vi "Connection Generator.vi"() -> ()   [LabVIEW 2019]
uses:
  <vilib>/numeric/Random Number (Range) I64.vi
  <vilib>/numeric/sub_Random U32.vi
panel:
  out "bytes written":i32
  out "error out (no error) 2":errorcluster
  in  "error in (no error)":errorcluster
  out "T1A1/A2":bool
  out "T1A13/A14":bool
  out "T1A11/A12":bool
  out "T1A9/A10":bool
  out "T1A8":bool
  out "T1A7":bool
  out "T1A5/A6":bool
  out "T1A3/A4":bool
  out "T1F3":bool
  out "T1F1/F2":bool
  out "T1E13/E14":bool
  out "T1E11/E12":bool
  out "T1E9/E10":bool
  out "T1E8":bool
  out "T1E7":bool
  out "T1E5":bool
  out "T1E3/E4":bool
  out "T1E1/E2":bool
  out "T1D13/D14":bool
  out "T1D11/D12":bool
  out "T1D9/D10":bool
  out "T1D8":bool
  out "T1D7":bool
  out "T1D5/D6":bool
  out "T1D3/D4":bool
  out "T1D1/D2":bool
  out "T1C13/C14":bool
  out "T1C11/C12":bool
  out "T1C9/C10":bool
  out "T1C8":bool
  out "T1C7":bool
  out "T1C5/C6":bool
  out "T1C3/C4":bool
  out "T1C1/C2":bool
  out "T1B13/B14":bool
  out "T1B11/B12":bool
  out "T1B9/B10":bool
  out "T1B8":bool
  out "T1B7":bool
  out "T1B5/B6":bool
  out "T1B3/B4":bool
  out "T1B1/B2":bool
  out "T2A1/A2":bool
  out "T2A13/A13":bool
  out "T2A11/A12":bool
  out "T2A9/A10":bool
  out "T2A8":bool
  out "T2A7":bool
  out "T2A5/A6":bool
  out "T2A3/A4":bool
  out "T2G5/G6":bool
  out "T2G3/G4":bool
  out "T2G1/G2":bool
  out "T2F6/F7":bool
  out "T2F4/F5":bool
  out "T2F3":bool
  out "T2F1/F2":bool
  out "T2E13/E14":bool
  out "T2E11/E12":bool
  out "T2E9/E10":bool
  out "T2E8":bool
  out "T2E7":bool
  out "T2E5/E6":bool
  out "T2E3/E4":bool
  out "T2E1/E2":bool
  out "T2D13/D14":bool
  out "T2D11/D12":bool
  out "T2D9/D10":bool
  out "T2D8":bool
  out "T2D7":bool
  out "T2D5/D6":bool
  out "T2D3/D4":bool
  out "T2D1/D2":bool
  out "T2C13/C14":bool
  out "T2C11/C12":bool
  out "T2C9/C10":bool
  out "T2C8":bool
  out "T2C7":bool
  out "T2C5/C6":bool
  out "T2C3/C4":bool
  out "T2C1/C2":bool
  out "T2B13/B14":bool
  out "T2B11/B12":bool
  out "T2B9/B10":bool
  out "T2B8":bool
  out "T2B7":bool
  out "T2B5/B6":bool
  out "T2B3/B4":bool
  out "T2B1/B2":bool
  out "I3":bool
  out "I2":bool
  out "I1":bool
  out "T3H6":bool
  out "T3H4":bool
  out "T3H3":bool
  out "T3H1":bool
  out "T3G13/G14":bool
  out "T3G11/G12":bool
  out "T3G9/G10":bool
  out "T3G8":bool
  out "T3G7":bool
  out "T3G5/G6":bool
  out "T3G3/G4":bool
  out "T3G1/G2":bool
  out "T3F13/F14":bool
  out "T3F11/F12":bool
  out "T3F9/F10":bool
  out "T3F8":bool
  out "T3F7":bool
  out "T3F5/F6":bool
  out "T3F3/F4":bool
  out "T3F1/F2":bool
  out "T3E13/E14":bool
  out "T3E11/E12":bool
  out "T3E9/E10":bool
  out "T3E8":bool
  out "T3E7":bool
  out "T3E5/E6":bool
  out "T3E3/E4":bool
  out "T3E1/E2":bool
  out "T3D13/D14":bool
  out "T3D11/D12":bool
  out "T3D9/D10":bool
  out "T3D8":bool
  out "T3D7":bool
  out "T3D5/D6":bool
  out "T3D3/D4":bool
  out "T3D1/D2":bool
  out "T3C13/C14":bool
  out "T3C11/C12":bool
  out "T3C9/C10":bool
  out "T3C8":bool
  out "T3C7":bool
  out "T3C5/C6":bool
  out "T3C3/C4":bool
  out "T3C1/C2":bool
  out "T3B13/B14":bool
  out "T3B11/B12":bool
  out "T3B9/B10":bool
  out "T3B8":bool
  out "T3B7":bool
  out "T3B5/B6":bool
  out "T3B3/B4":bool
  out "T3B1/B2":bool
  out "T3A13/A14":bool
  out "T3A11/A12":bool
  out "T3A9/A10":bool
  out "T3A8":bool
  out "T3A7":bool
  out "T3A5/A6":bool
  out "T3A3/A4":bool
  out "T3A1/A2":bool
  in  "Stop":bool
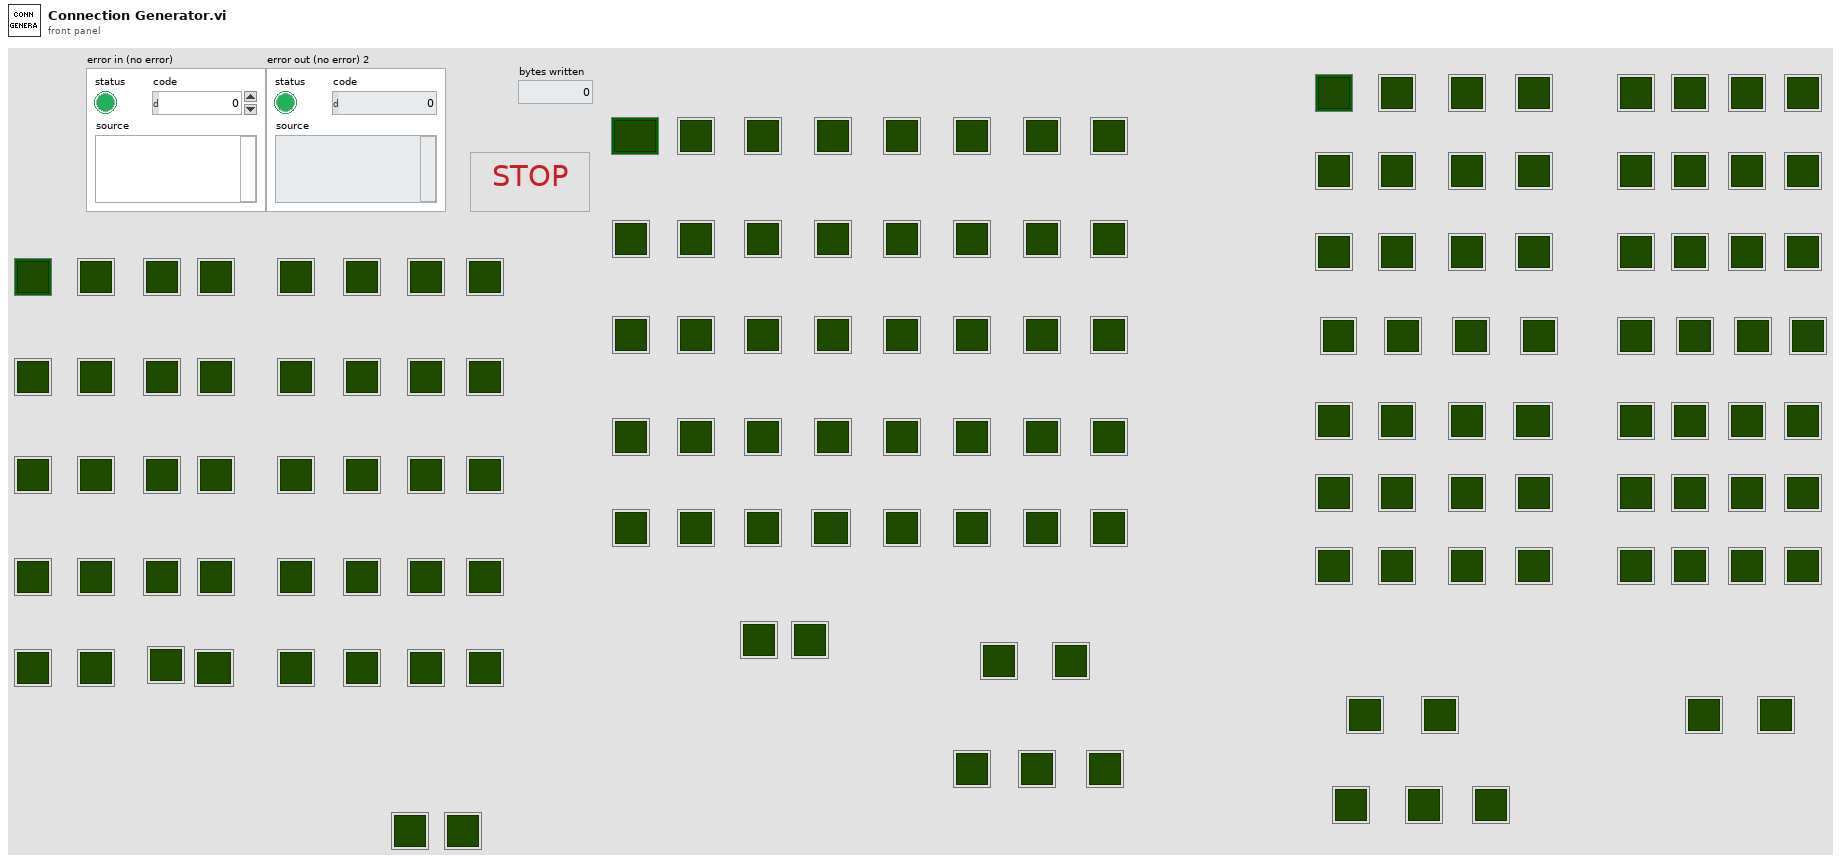
[diagram p1: front panel]
types:
  T1 = enum16{"Initialize", "Create Random String", "Open Connection", "Send Data", "Close Connection", "Exit"}
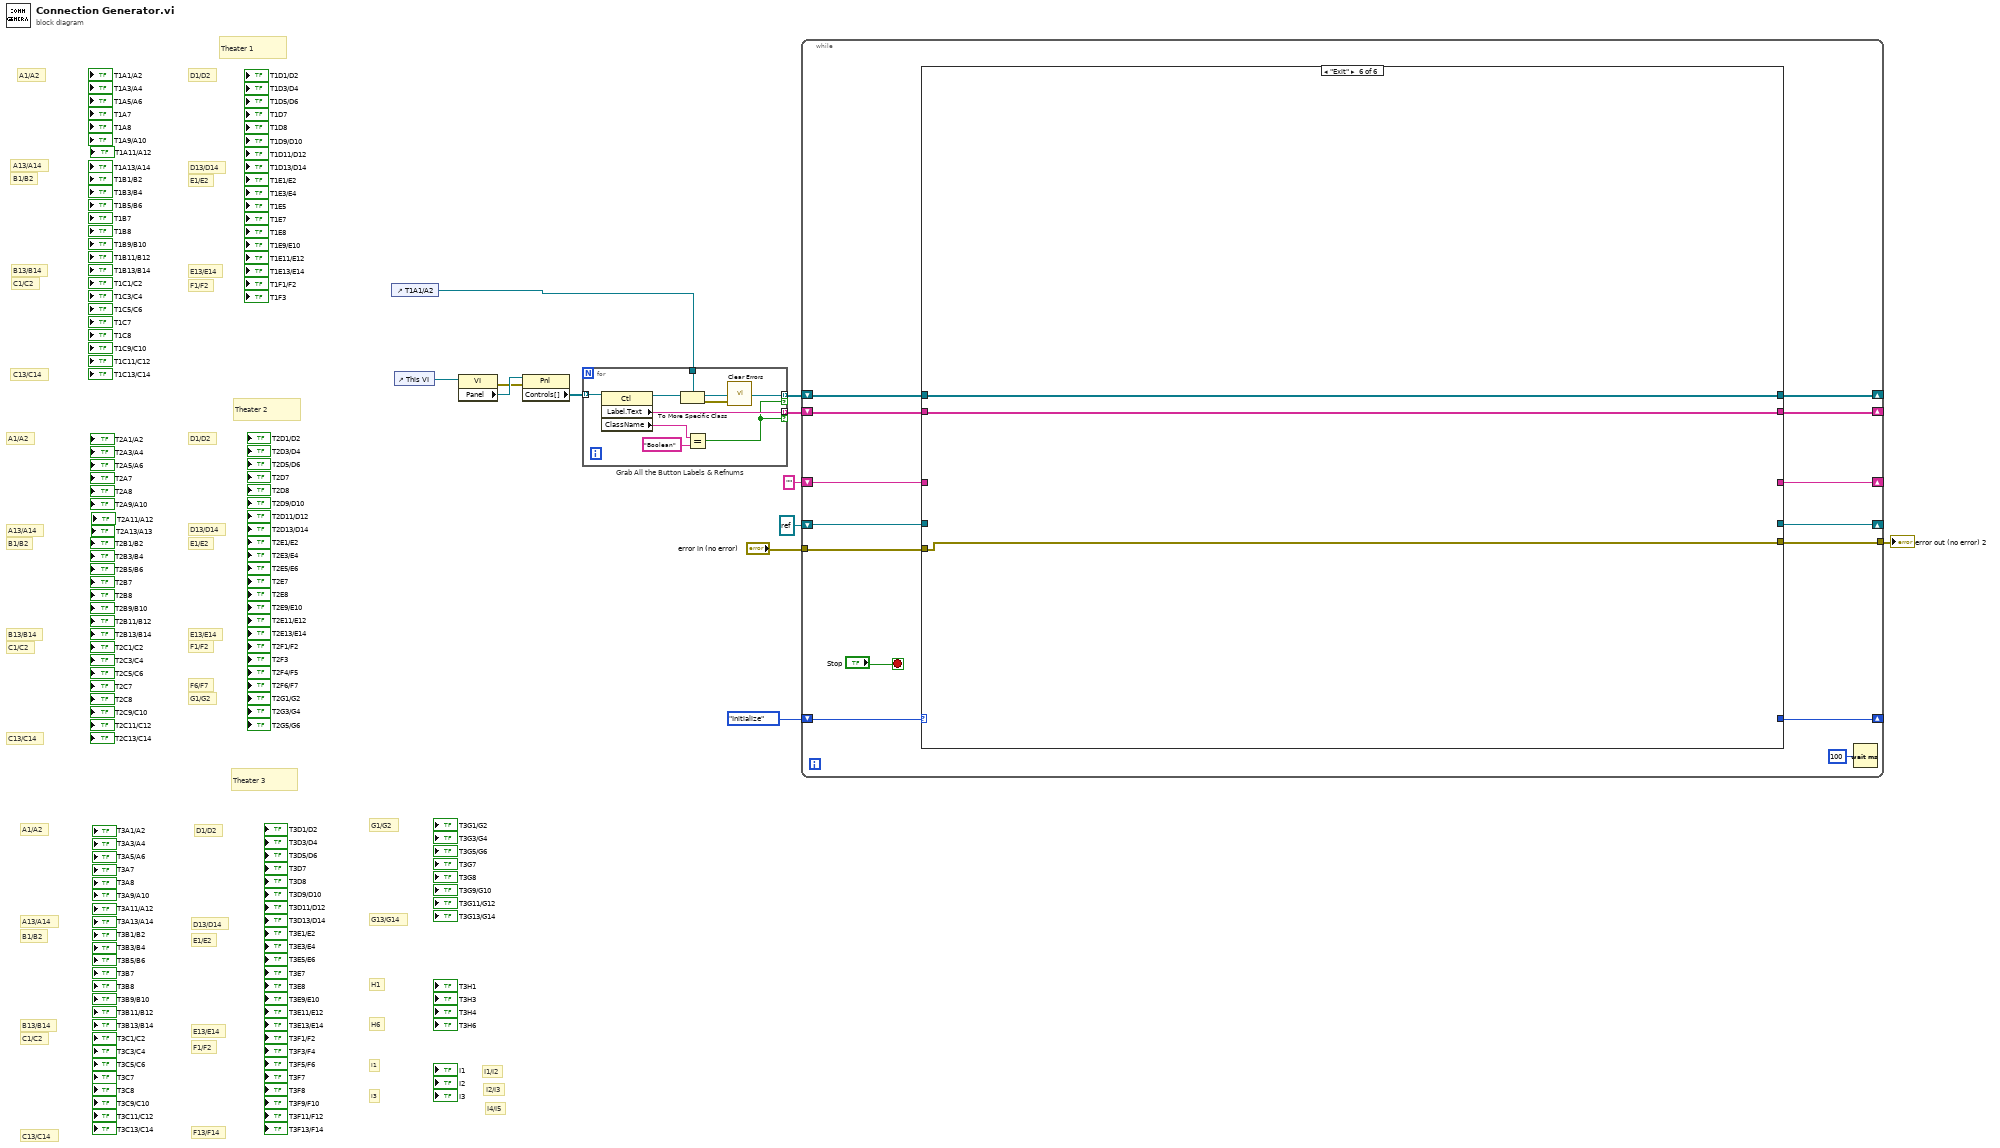
[diagram p0: block diagram]
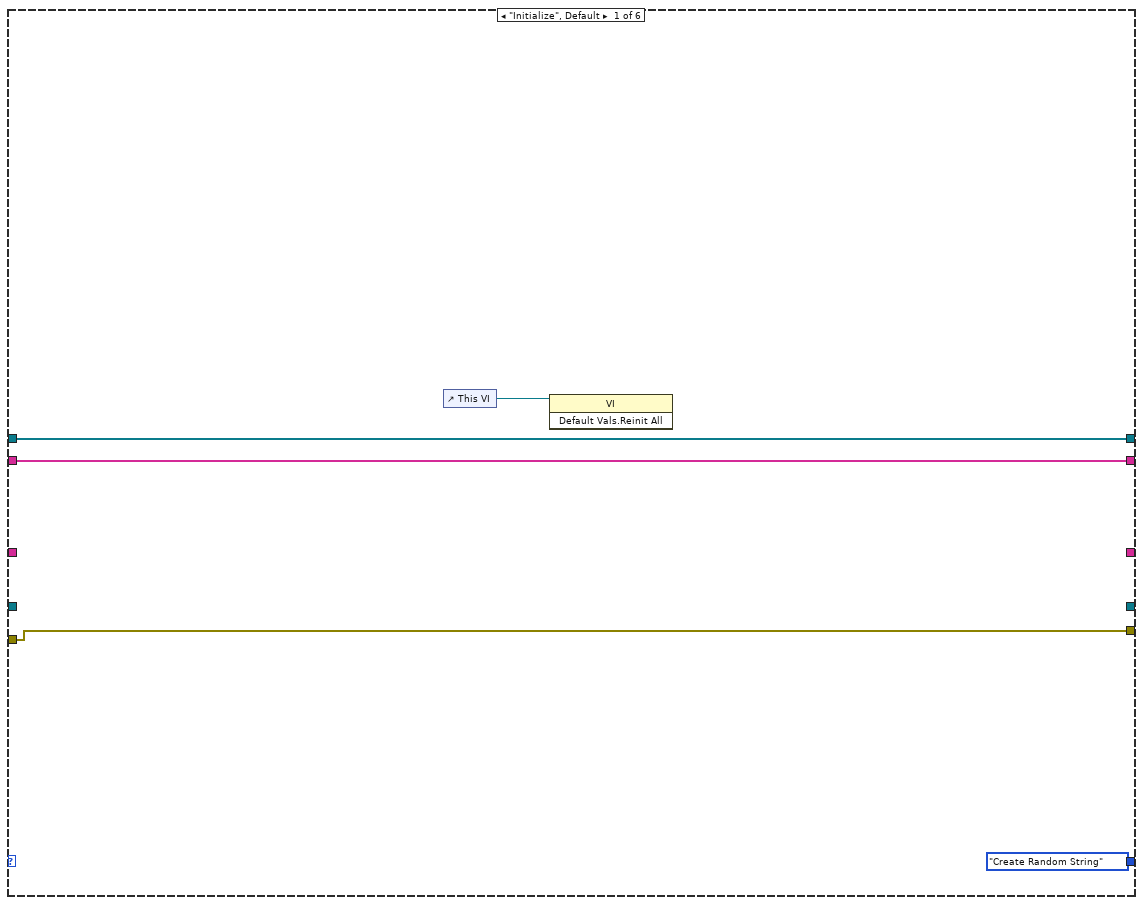
[diagram p2: hidden frame]
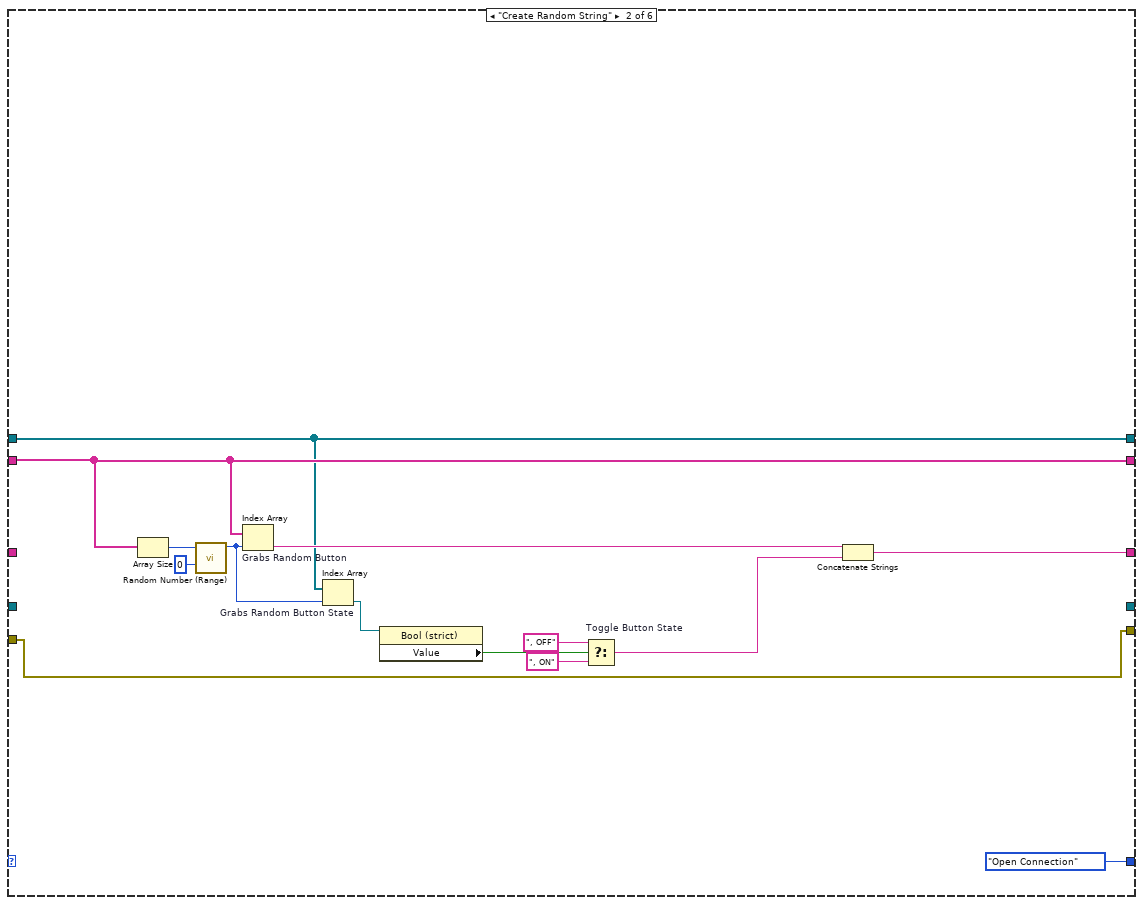
[diagram p3: hidden frame]
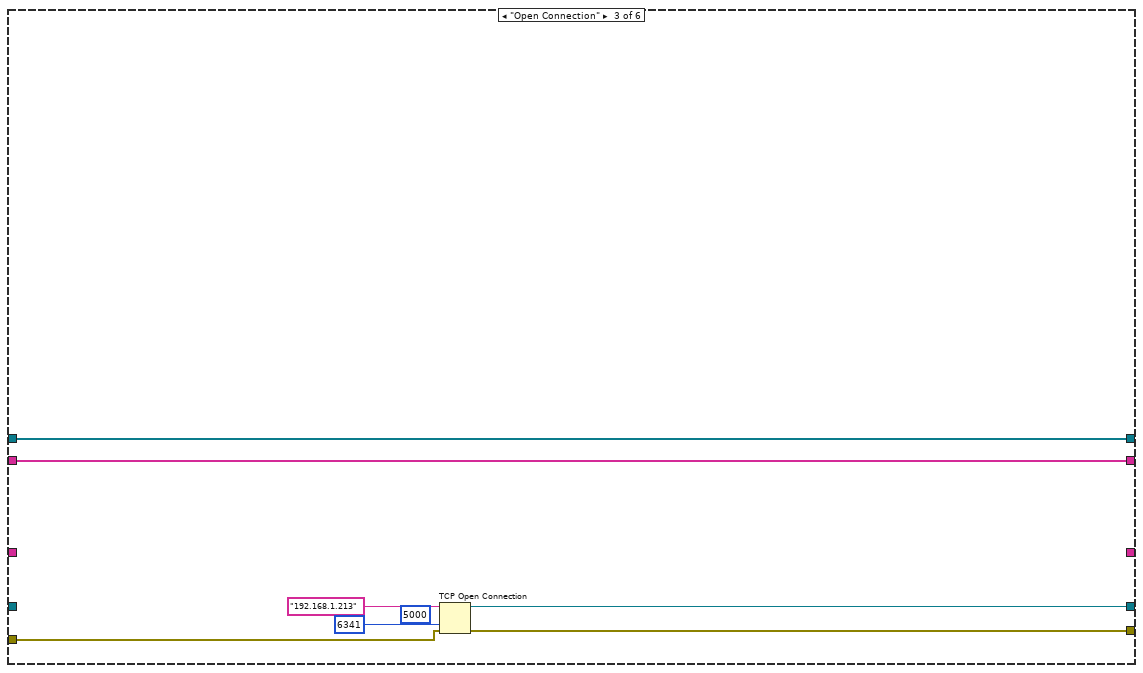
[diagram p4: hidden frame]
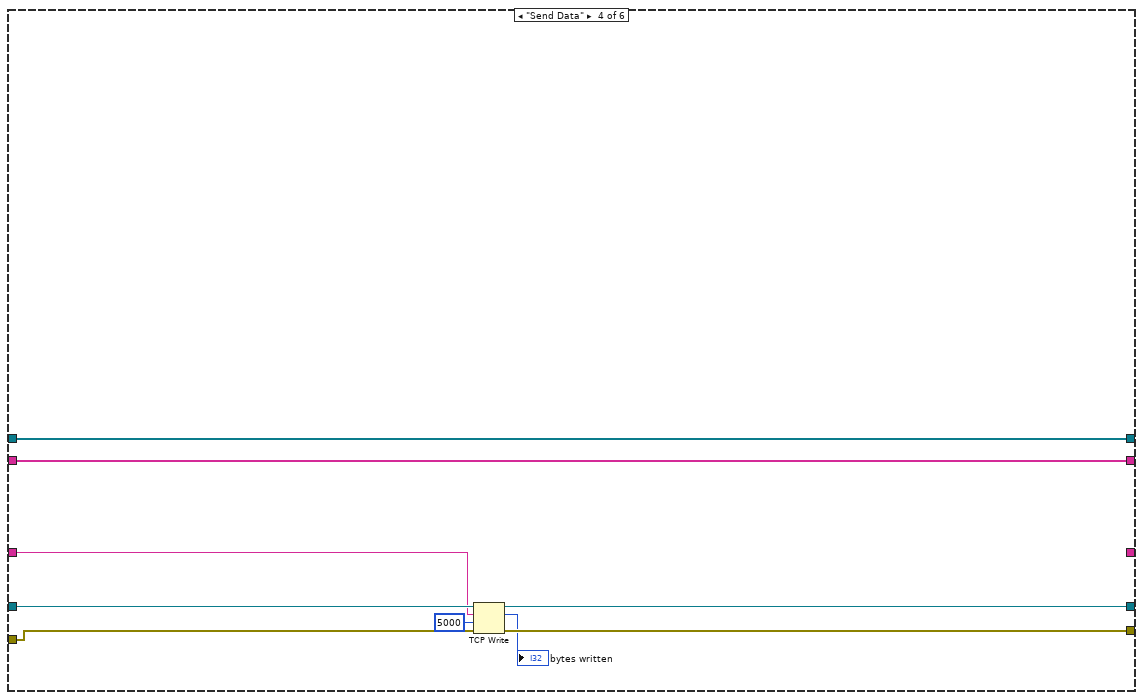
[diagram p5: hidden frame]
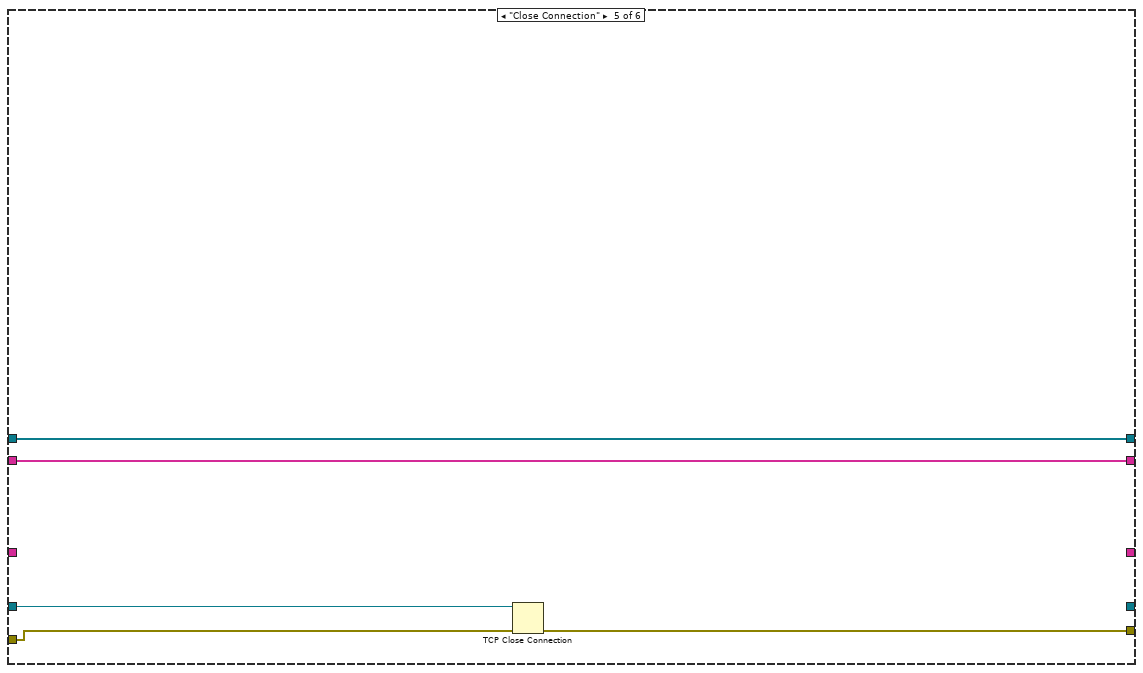
[diagram p6: hidden frame]
diagram:
  # "I4/I5"
  # "I2/I3"
  # "I1/I2"
  # "C13/C14"
  # "C1/C2"
  # "B13/B14"
  # "B1/B2"
  # "A13/A14"
  # "F1/F2"
  # "E13/E14"
  # "E1/E2"
  # "D1/D2"
  # "D13/D14"
  # "A1/A2"
  # "Theater 1"
  # "G1/G2"
  # "F6/F7"
  # "F1/F2"
  # "E13/E14"
  # "C13/C14"
  # "C1/C2"
  # "B13/B14"
  # "E1/E2"
  # "D1/D2"
  # "D13/D14"
  # "B1/B2"
  # "A13/A14"
  # "A1/A2"
  # "Theater 2"
  # "G13/G14"
  # "H6"
  # "I3"
  # "I1"
  # "H1"
  # "G1/G2"
  # "F13/F14"
  # "F1/F2"
  # "E13/E14"
  # "E1/E2"
  # "D1/D2"
  # "D13/D14"
  # "C13/C14"
  # "C1/C2"
  # "B13/B14"
  # "B1/B2"
  # "A13/A14"
  # "A1/A2"
  # "Theater 3"
  n1 = control-ref of="T1A1/A2"() -> (w8:refnum<vi>)
  n2 = control-ref of="This VI"() -> (w12:refnum<vi>)
  n3 = property class="VI"(reference=w12) -> (error out=w10:errorcluster, "Panel"=w11:refnum<vi>)  [unwired: 1 in, 1 out]
  n4 = property class="Pnl"(reference=w11, error in=w10) -> ("Controls[]"=w9:refnum<vi>[])  [unwired: 2 out]
  n5 = for "Grab All the Button Labels & Refnums" {
    tunnel: w9 -> [w21] mode=indexing
    tunnel: [w14] -> w7 mode=indexing if=w17
    tunnel: [w18] -> w6 mode=indexing if=w17
    tunnel: w8 -> [w15]
    n6 = property class="Ctl"(reference=w21) -> (reference out=w16:refnum<vi>, "Label.Text"=w18:string, "ClassName"=w19:string)  [unwired: 1 in, 1 out]
    n7 = To More Specific Class(target class=w15, reference=w16) -> (specific class reference=w14:refnum<vi>, error out=w13:errorcluster)  [unwired: 1 in]
    n8 = Equal?(x=w19, y="Boolean" ("regular expression")) -> (x = y?=w17:bool)
    n9 = call <vilib>:"Clear Errors.vi"("error in (no error)"=w13) -> ()  [unwired: 5 in, 2 out]
  }
  n10 = while {
    shift-right: [w28] -> _
    shift-left: w7 -> [w30]
    shift-right: [w29] -> _
    shift-left: w6 -> [w31]
    shift-right: [w32] -> _
    shift-left: T1."Initialize" -> [w33]
    shift-right: [w27] -> _
    shift-left: "" -> [w26]
    tunnel: "error in (no error)" -> [w25]
    tunnel: [w24] -> w2
    shift-right: [w23] -> _
    shift-left: refnum<k5> refnum ("connection ID") -> [w22]
    stop <- "Stop" stop-if-true
    n11 = case shown="\"Exit\"" w33 {
      tunnel: [T1."Create Random String" T1."Open Connection" _ _ _ _] -> w32
      tunnel: w31 -> [w38 w52 w60 w69 w74 w77]
      tunnel: w30 -> [w39 w46 w61 w70 w75 w78]
      tunnel: [w38 w52 w60 w69 w74 w77] -> w29
      tunnel: [w39 w46 w61 w70 w75 w78] -> w28
      tunnel: [_ w43 _ _ _ _] -> w27
      tunnel: w26 -> [_ _ _ w64 _ _]
      tunnel: w25 -> [w36 w41 w57 w67 w71 w76]
      tunnel: [w36 w41 w56 w68 w72 w76] -> w24
      tunnel: [_ _ w55 w62 _ _] -> w23
      tunnel: w22 -> [_ _ _ w66 w73 _]
      frame "Initialize", Default {
        n12 = control-ref of="This VI"() -> (w40:refnum<vi>)
        n13 = invoke class="VI" method="Default Vals.Reinit All"(reference=w40) -> ()  [unwired: 2 in, 3 out]
      }
      frame "Create Random String" {
        n14 = Array Size(array=w52) -> (size(s)=w54:i32)
        n15 = call-poly <vilib>:"Random Number (Range).vi"("lower bound (-100)"=i64 0, "upper bound (100)"=w54) -> ("number"=w47:i64)  [unwired: 9 in]
        n16 = Index Array "Grabs Random Button"(array=w52, index=w47) -> (element=w49:string)
        n17 = Index Array "Grabs Random Button State"(array=w46, index=w47) -> (element=w45:refnum<vi>)
        n18 = property class="Bool (strict)"(reference=w45) -> ("Value"=w44:bool)  [unwired: 1 in, 2 out]
        n19 = Select "Toggle Button State"(t=", OFF", s=w44, f=", ON") -> (s? t:f=w48:string)
        n20 = Concatenate Strings(w49, w48) -> (w43:string)
      }
      frame "Open Connection" {
        (unwired) u16 5000 ("remote port or service name")
        n21 = TCP Open Connection(address="192.168.1.213", remote port or service name=u16 6341, error in (no error)=w57) -> (connection ID=w55:refnum<k5>, error out=w56:errorcluster)  [unwired: 2 in]
      }
      frame "Send Data" {
        n22 = TCP Write(connection ID=w66, data in=w64, error in (no error)=w67, 9:5000 ("timeout ms (25000)")) -> (connection ID out=w62:refnum<k5>, bytes written=→"bytes written":i32, error out=w68:errorcluster)
      }
      frame "Close Connection" {
        n23 = TCP Close Connection(connection ID=w73, error in (no error)=w71) -> (error out=w72:errorcluster)  [unwired: 1 in, 1 out]
      }
      frame "Exit" {
      }
    }
    n24 = Wait (ms)(milliseconds to wait=u32 100) -> ()  [unwired: 1 out]
  }
  "error out (no error) 2" <- w2
